vi "Check for Names v2.vi"(0 "New Name":string, 1 "Name List":string[](array[string]), 2 "Empty Plots?":bool[](array[boolean]), 3 "Error In":errorcluster, 4 "Suffix Format String (<Space>%d)":string=" %d") -> (5 "New Name List":string[](array[string]), 6 "New Name":string, 7 "Checked Array":bool[](array[boolean]), 9 "Error Out":errorcluster)   [LabVIEW 2019]
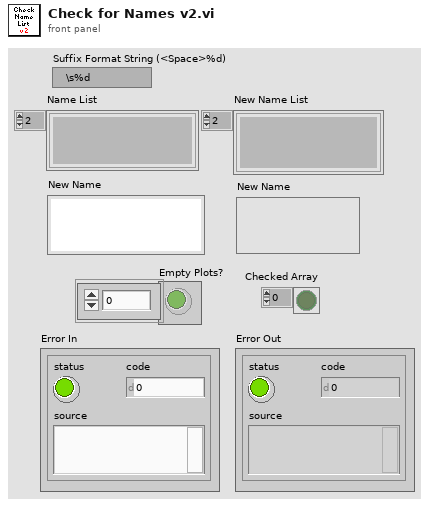
[diagram p1: front panel]
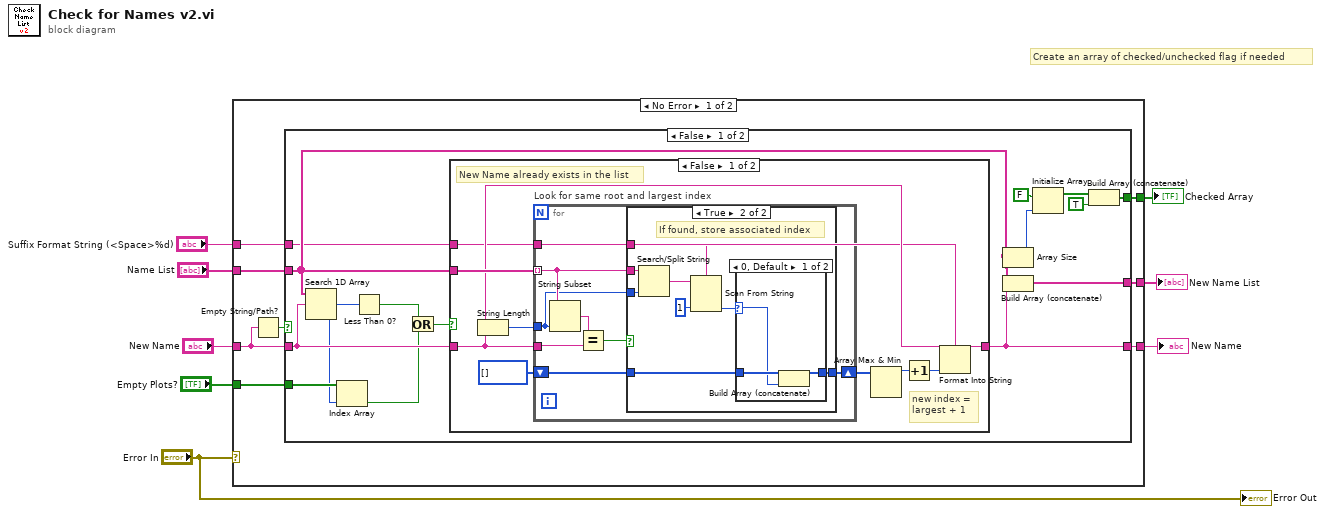
[diagram p0: block diagram]
diagram:
  # "Create an array of checked/unchecked flag if needed"
  n1 = case shown="No Error" "Error In" {
    tunnel: [w16 w65] -> w8
    tunnel: [w15 w66] -> w7
    tunnel: [w14 _] -> w6
    tunnel: "Name List" -> [w13 w66]
    tunnel: "New Name" -> [w12 w65]
    tunnel: "Empty Plots?" -> [w10 _]
    tunnel: "Suffix Format String (<Space>%d)" -> [w9 _]
    frame No Error {
      n2 = Empty String/Path?(string/path=w12) -> (empty?=w11:bool)
      n3 = case shown="False" w11 {
        tunnel: [w31 w63] -> w16
        tunnel: [w30 w64] -> w15
        tunnel: [w25 _] -> w14
        tunnel: w13 -> [w24 w64]
        tunnel: w12 -> [w23 w63]
        tunnel: w10 -> [w22 _]
        tunnel: w9 -> [w17 _]
        frame False {
          n4 = Search 1D Array(1D array=w24, element=w23) -> (index of element=w21:i32)  [unwired: 1 in]
          n5 = Index Array(array=w22, index=w21) -> (element=w19:bool)
          n6 = Less Than 0?(x=w21) -> (x < 0?=w20:bool)
          n7 = Or(x=w20, y=w19) -> (x .or. y?=w18:bool)
          n8 = case shown="False" w18 {
            tunnel: w23 -> [w33 w62]
            tunnel: [w35 w62] -> w31
            tunnel: w24 -> [w40 _]
            tunnel: w17 -> [w32 _]
            frame False {
              # "new index =\nlargest + 1"
              # "New Name already exists in the list"
              n9 = String Length(string=w33) -> (length=w34:i32)
              n10 = for "Look for same root and largest index" {
                tunnel: w40 -> [w43] mode=indexing
                tunnel: w33 -> [w45]
                shift-right: [w47] -> w38
                shift-left: i32[] [] -> [w48]
                tunnel: w34 -> [w42]
                tunnel: w32 -> [w41]
                n11 = String Subset(string=w43, length (rest)=w42) -> (substring=w46:string)  [unwired: 1 in]
                n12 = Equal?(x=w46, y=w45) -> (x = y?=w44:bool)
                n13 = case shown="True" w44 {
                  tunnel: w48 -> [w49 w56]
                  tunnel: [w49 w55] -> w47
                  tunnel: w43 -> [_ w54]
                  tunnel: w42 -> [_ w53]
                  tunnel: w41 -> [_ w50]
                  frame False {
                  }
                  frame True {
                    # "If found, store associated index"
                    n14 = Search/Split String(string=w54, offset (0)=w53) -> (match + rest of string=w52:string)  [unwired: 1 in, 2 out]
                    n15 = Scan From String(format string=w50, input string=w52, default 1=1 ("Default Value 1")) -> (output 1=w51:i32)  [unwired: 2 in, 3 out]
                    n16 = case shown="0, Default" w51 {
                      selector: w51 -> [w58 _]
                      tunnel: w56 -> [w60 w61]
                      tunnel: [w59 w61] -> w55
                      frame 0, Default {
                        n17 = Build Array (concatenate)(w60, w58) -> (w59:i32[])
                      }
                      frame -1 {
                        # "not an index"
                      }
                    }
                  }
                }
              }
              n18 = Array Max & Min(array=w38) -> (max value=w37:i32)  [unwired: 3 out]
              n19 = Increment(x=w37) -> (x+1=w36:i32)
              n20 = Format Into String(format string=w32, initial string=w33, w36) -> (resulting string=w35:string)  [unwired: 1 in, 1 out]
            }
            frame True {
              # "New Name does not conflict with any existing ones\nor it is because the plot is empty"
            }
          }
          n21 = Array Size(array=w24) -> (size(s)=w29:i32)
          n22 = Build Array (concatenate)(w24, w31) -> (w30:string[])
          n23 = Initialize Array(FALSE, w29) -> (w27:bool[])
          n24 = Build Array (concatenate)(w27, TRUE ("Input Element")) -> (w25:bool[])
        }
        frame True {
        }
      }
    }
    frame Error {
    }
  }
  "New Name" <- w8
  "New Name List" <- w7
  "Checked Array" <- w6
  "Error Out" <- "Error In"
